vi "Configure Measurement (Burst).vi"(8 "error in (no error)":errorcluster, 10 "Burst Type (0: Positive Width Measurement)":i32(ring) items=["Positive Width Measurement", "Negative Width Measurement", "Frequency"], 11 "VISA resource name":refnum<visa-resource-name>) -> (0 "error out":errorcluster, 3 "VISA resource name out":refnum<visa-resource-name>)   [LabVIEW 2024, in "Agilent 532XX Series.lvlib"]
doc: "Configures the setting for the Burst\n\n<B>Notes:</B> \nThis VI only applies to the Agilent 53230A. \nRequires option 150 and takes all measurments on channel 3."
uses:
  Agilent 532XX Series.lvlib
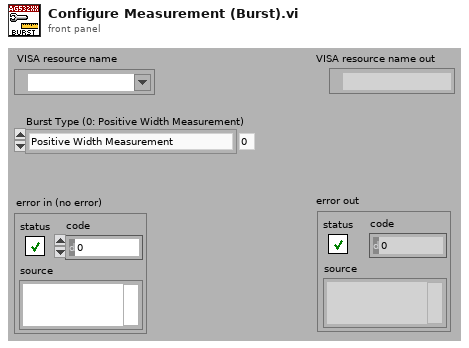
[diagram p1: front panel]
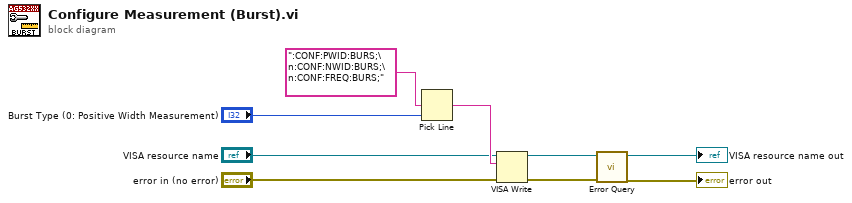
[diagram p0: block diagram]
diagram:
  n1 = Pick Line(multi-line string=":CONF:PWID:BURS;\n:CONF:NWID:BURS;\n:CONF:FREQ:BURS;", line index="Burst Type (0: Positive Width Measurement)") -> (output string=w7:string)  [unwired: 1 out]
  n2 = VISA Write(VISA resource name="VISA resource name", write buffer=w7, error in (no error)="error in (no error)") -> (VISA resource name out=w4:refnum<visa-resource-name>, error out=w3:errorcluster)  [unwired: 1 out]
  n3 = call "Error Query.vi"("error in (no error)"=w3, "VISA resource name"=w4) -> ("error out"=→"error out":errorcluster, "VISA resource name out"=→"VISA resource name out":refnum<visa-resource-name>)  [unwired: 8 out]
